vi "Set Vantage Tx Config V.vi"(8 "error in (no error)":errorcluster, 11 "txConfig":T1) -> (0 "error out":errorcluster, 2 "function return":i16, 3 "txConfig out":T1)   [LabVIEW 2009, in "VantagePro.lvlib"]
doc: "DllAccess short int _stdcall SetVantageTxConfig_V ( TxConfiguration *txConfig);"
uses:
  VantagePro.lvlib
  <userlib>/VantagePro/VantagePro.dll
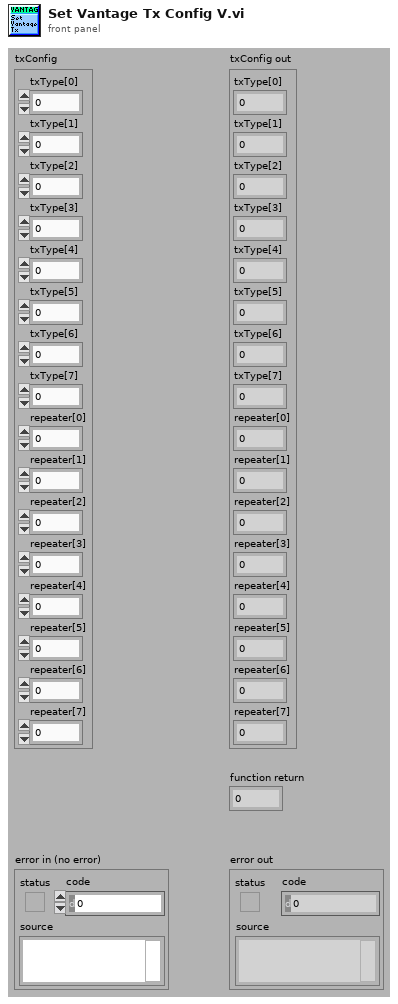
[diagram p1: front panel]
types:
  T1 = cluster{"txType[0]":i16, "txType[1]":i16, "txType[2]":i16, "txType[3]":i16, "txType[4]":i16, "txType[5]":i16, "txType[6]":i16, "txType[7]":i16, "repeater[0]":i16, "repeater[1]":i16, "repeater[2]":i16, "repeater[3]":i16, "repeater[4]":i16, "repeater[5]":i16, "repeater[6]":i16, "repeater[7]":i16}
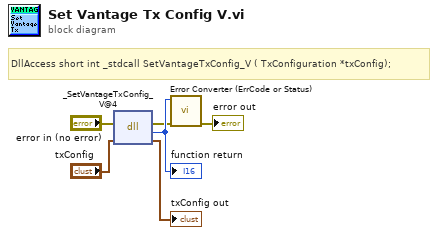
[diagram p0: block diagram]
diagram:
  # "DllAccess short int _stdcall SetVantageTxConfig_V ( TxConfiguration *txConfig);"
  n1 = dll-call lib="C:/Program Files/National Instruments/LabVIEW 2010/user.lib/VantagePro/VantagePro.*" fn="_SetVantageTxConfig_V@4"(error in="error in (no error)", "txConfig"="txConfig") -> (error out=w2:errorcluster, w6:i16, "txConfig"=→"txConfig out":T1)  [unwired: 2 in, 1 out]
  "function return" <- w6
  n2 = call "Error Converter (ErrCode or Status).vi"("error in (no error)"=w2, "error code"=w6) -> ("error out"=→"error out":errorcluster)  [unwired: 9 in]
